vi "libssh2_userauth_banner.vi"(8 "error in (no error)":errorcluster, 11 "session":T1) -> (0 "error out":errorcluster, 2 "banner":string, 3 "return value":i32)   [LabVIEW 2013, in "libssh2.lvlib"]
doc: "Gets the server's userauth banner message."
uses:
  libssh2.lvlib
  Session Refnum.ctl
  libssh2.dll
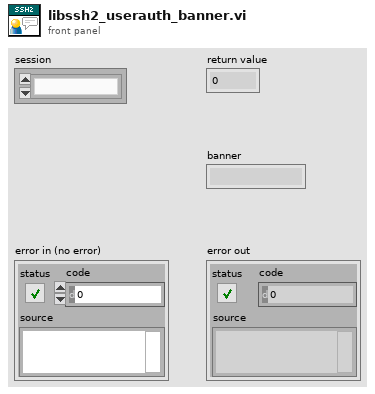
[diagram p1: front panel]
types:
  T1 = typedef "libssh2.lvlib/Session Refnum.ctl" = refnum<k1>
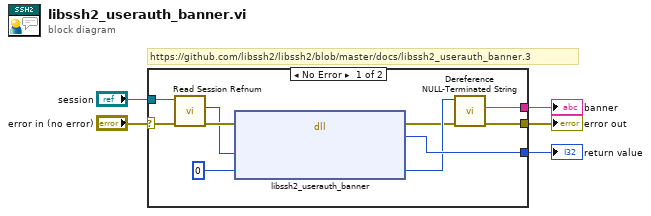
[diagram p0: block diagram]
diagram:
  # "https://github.com/libssh2/libssh2/blob/master/docs/libssh2_userauth_banner.3"
  n1 = case shown="No Error" "error in (no error)" {
    selector: "error in (no error)" -> [w9 w16]
    tunnel: [w15 _] -> w5
    tunnel: [w6 w16] -> w4
    tunnel: [w13 _] -> w3
    tunnel: "session" -> [w11 _]
    frame No Error {
      n2 = call "Read Session Refnum.vi"("error in (no error)"=w9, "session"=w11) -> ("error out"=w12:errorcluster, "LIBSSH2_SESSION*"=w10:u64)  [unwired: 8 in]
      n3 = dll-call lib="C:/Users/pasca/source/repos/libssh2-labview/libssh2**.*" fn="libssh2_userauth_banner"(error in=w12, "session"=w10, "banner"=u64 0) -> (error out=w7:errorcluster, "return value"=w15:i32, "banner"=w8:u64)  [unwired: 3 in, 1 out]
      n4 = call "Dereference NULL-Terminated String.vi"("error in (no error)"=w7, "char*"=w8) -> ("error out"=w6:errorcluster, "string"=w13:string)  [unwired: 8 in]
    }
    frame Error {
    }
  }
  "return value" <- w5
  "error out" <- w4
  "banner" <- w3
